vi "User Shell.vi"() -> ()   [LabVIEW 2014]
panel:
  in  "file path (use dialog)":path
  in  "Exit":bool
  in  "Cluster":T1
  in  "Run":bool
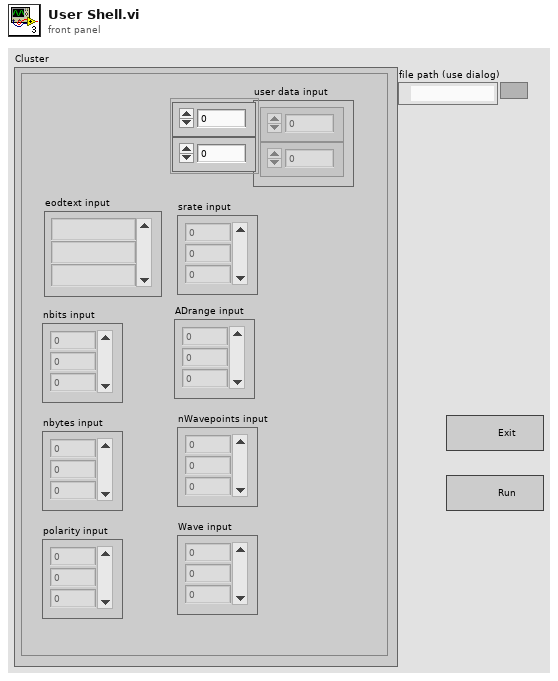
[diagram p1: front panel]
types:
  T1 = cluster{"eodtext input":string[], "nbits input":i8[], "nbytes input":i8[], "polarity input":i8[], "user data input":sgl[][], "srate input":u32[], "ADrange input":sgl[], "nWavepoints input":u32[], "Wave input":i16[]}
  T2 = enum16{"Run", "Wait", "Change value", "Exit", "Display message"}
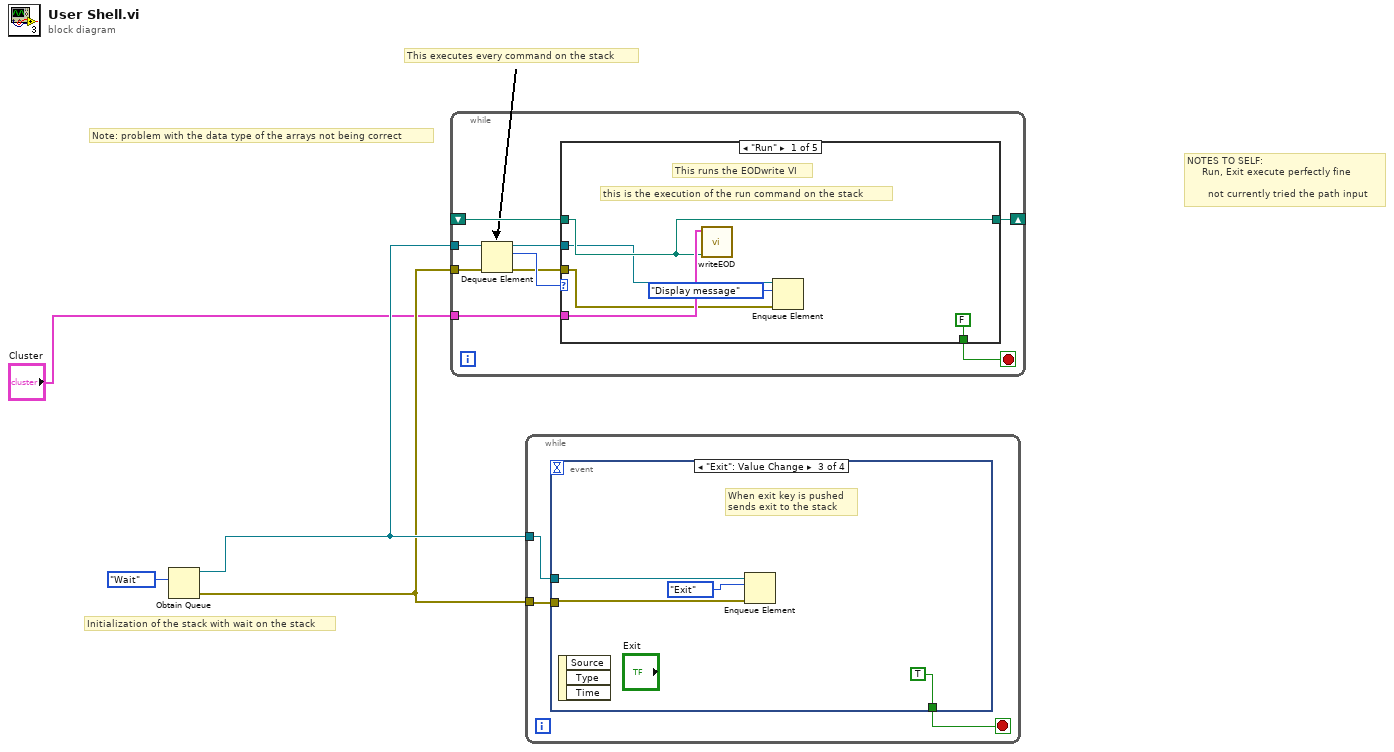
[diagram p0: block diagram]
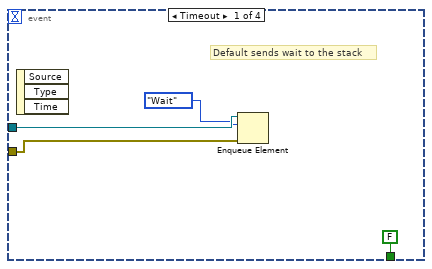
[diagram p2: hidden frame]
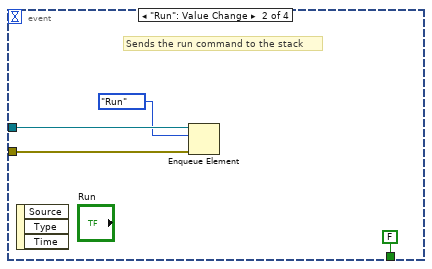
[diagram p3: hidden frame]
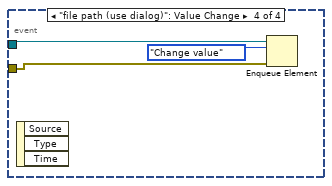
[diagram p4: hidden frame]
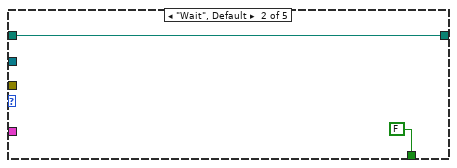
[diagram p5: hidden frame]
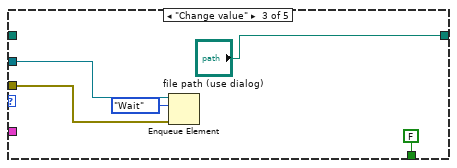
[diagram p6: hidden frame]
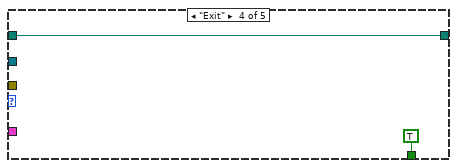
[diagram p7: hidden frame]
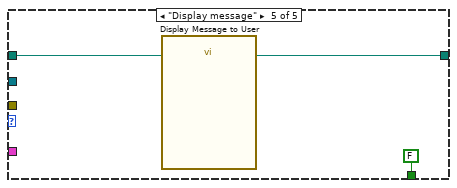
[diagram p8: hidden frame]
diagram:
  # "NOTES TO SELF:\n     Run, Exit execute perfectly fine\n\n       not currently tried the path input"
  # "Initialization of the stack with wait on the stack"
  # "This executes every command on the stack"
  # "Note: problem with the data type of the arrays not being correct"
  n1 = Obtain Queue(element data type=T2."Wait") -> (queue out=w3:refnum<queue>, error out=w2:errorcluster)  [unwired: 4 in, 1 out]
  n2 = while {
    tunnel: w3 -> [w12]
    tunnel: w2 -> [w11]
    tunnel: "Cluster" -> [w9]
    shift-right: [w8] -> _
    shift-left: _ -> [w7]
    stop <- w13 stop-if-true
    n3 = Dequeue Element(queue=w12, error in (no error)=w11) -> (queue out=w6:refnum<queue>, element=w10:T2, error out=w5:errorcluster)  [unwired: 1 in, 1 out]
    n4 = case shown="\"Run\"" w10 {
      tunnel: [FALSE FALSE FALSE TRUE FALSE] -> w13
      tunnel: w9 -> [w18 _ _ _ _]
      tunnel: [w17 w20 "file path (use dialog)" w27 w29] -> w8
      tunnel: w7 -> [w17 w20 _ w27 w29]
      tunnel: w6 -> [w16 _ w24 _ _]
      tunnel: w5 -> [w15 _ w23 _ _]
      frame "Run" {
        # "this is the execution of the run command on the stack"
        # "This runs the EODwrite VI"
        n5 = call "writeEOD.vi"("file path (use dialog)"=w17, "Cluster"=w18) -> ()  [unwired: 8 in, 2 out]
        n6 = Enqueue Element(queue=w16, element=T2."Display message", error in (no error)=w15) -> ()  [unwired: 1 in, 3 out]
      }
      frame "Wait", Default {
      }
      frame "Change value" {
        n7 = Enqueue Element(queue=w24, element=T2."Wait", error in (no error)=w23) -> ()  [unwired: 1 in, 3 out]
      }
      frame "Exit" {
      }
      frame "Display message" {
        n8 = call "Display Message to User"() -> ()  [unwired: 10 in, 2 out]
      }
    }
  }
  n9 = while {
    tunnel: w3 -> [w33]
    tunnel: w2 -> [w32]
    stop <- w31 stop-if-true
    n10 = event shown="[2] \"Exit\": Value Change" {
      selector: _ -> [_ _ _ _]
      dyn-events: _ -> [_ _ _ _]
      timeout: _ -> [_ _ _ _]
      tunnel: w33 -> [w37 w41 w44 w47]
      tunnel: w32 -> [w36 w40 w43 w46]
      tunnel: [FALSE FALSE TRUE _] -> w31
      event Timeout {
        # "Default sends wait to the stack"
        n11 = event-data() -> ()  [unwired: 1 in, 3 out]
        n12 = Enqueue Element(queue=w37, element=T2."Wait", error in (no error)=w36) -> ()  [unwired: 1 in, 3 out]
      }
      event "Run": Value Change {
        # "Sends the run command to the stack"
        n13 = event-data() -> ()  [unwired: 1 in, 3 out]
        n14 = Enqueue Element(queue=w41, element=T2."Run", error in (no error)=w40) -> ()  [unwired: 1 in, 3 out]
      }
      event "Exit": Value Change {
        # "When exit key is pushed\nsends exit to the stack"
        n15 = event-data() -> ()  [unwired: 1 in, 3 out]
        n16 = Enqueue Element(queue=w44, element=T2."Exit", error in (no error)=w43) -> ()  [unwired: 1 in, 3 out]
      }
      event "file path (use dialog)": Value Change {
        n17 = event-data() -> ()  [unwired: 1 in, 3 out]
        n18 = Enqueue Element(queue=w47, element=T2."Change value", error in (no error)=w46) -> ()  [unwired: 1 in, 3 out]
      }
    }
  }
